vi "Measure_Synthetic_Jet.vi"(3 "Mode":T1=enum."Run VI", 5 "Traverse line In":T3={"Start X"=0.0, "Start Y"=0.0, "Start Z"=0.0, "End X"=nan, "End Y"=nan, "End Z"=nan, "nPoints"=5, "Spacing"=enum."Linear", "Filename"=path "C:/EnFlo_Data_Local/2013/Aero_Tunnel/Nick_Martin/Results/01-2013/QA_test_I.xls", "Tunnel Speed"=nan, "Averaging time (mins)"=0.08, "Extra Commands"="", "Carrier_1 Q (l/min)"=nan, "Carrier_2 Q (l/min)"=5.0, "Trace Gas Concentration (%)"=nan, "Specific Arguments"="Measure_Synthetic_Jet.vi; 200; 1000; 100", "Comments"="", "Row No"=0, "Row Type Selector"=enum."Run VI Named:", "EstCompl"="17:12  07-01-2013", "Row Duration (mins)"=4.483248000000001, "nValidPoints"=5, "Meas Setup File"="LDA_SJ_A.xls"} {"Carrier_2 Q (l/min)" format="%#.2f"; "Row Duration (mins)" format="%#.1f"; "Row No" min=0; "Trace Gas Concentration (%)" min=0.0 format="%#_4f"; "Carrier_1 Q (l/min)" format="%#.4f"; "Start X" format="%#.2f"; "Start Y" format="%#.2f"; "Start Z" format="%#.2f"; "End X" format="%#.2f"; "End Y" format="%#.2f"; "End Z" format="%#.2f"; "Tunnel Speed" format="%#.2f"; "Averaging time (mins)" min=0.0 format="%#.2f"}) -> (0 "Error Message":string, 1 "Status":T2, 2 "Traverse line Out":T3={"Start X"=0.0, "Start Y"=0.0, "Start Z"=0.0, "End X"=nan, "End Y"=nan, "End Z"=nan, "nPoints"=5, "Spacing"=enum."Linear", "Filename"=path "C:/EnFlo_Data_Local/2013/Aero_Tunnel/Nick_Martin/Results/01-2013/QA_test_I.xls", "Tunnel Speed"=nan, "Averaging time (mins)"=0.08, "Extra Commands"="", "Carrier_1 Q (l/min)"=nan, "Carrier_2 Q (l/min)"=5.0, "Trace Gas Concentration (%)"=nan, "Specific Arguments"="Measure_Synthetic_Jet.vi; 200; 1000; 100", "Comments"="", "Row No"=0, "Row Type Selector"=enum."Run VI Named:", "EstCompl"="17:12  07-01-2013", "Row Duration (mins)"=4.483248000000001, "nValidPoints"=5, "Meas Setup File"="LDA_SJ_A.xls"} {"Carrier_2 Q (l/min)" format="%#.2f"; "Row Duration (mins)" format="%#.1f"; "Row No" min=0; "Trace Gas Concentration (%)" min=0.0 format="%#_4f"; "Carrier_1 Q (l/min)" format="%#.4f"; "Start X" format="%#.2f"; "Start Y" format="%#.2f"; "Start Z" format="%#.2f"; "End X" format="%#.2f"; "End Y" format="%#.2f"; "End Z" format="%#.2f"; "Tunnel Speed" format="%#.2f"; "Averaging time (mins)" min=0.0 format="%#.2f"})   [LabVIEW 2022 SP3]
uses:
  <vilib>/Analysis/NI_AALBase.lvlib
  Globals/Synthetic_jet_global.vi
  Controls/Setup.ctl
  Controls/Save_Data.ctl
  Globals/Extra_Commands_Global.vi
  ADAM Client/Sub VIs/ADAM Controls/Update_scan_value.ctl
  <vilib>/Analysis/1siggen.llb/Ramp Pattern by Samples.vi
  Globals/Meas_global.vi
  Controls/User_Specific_mode.ctl
  Gen Trav/Multi_Run_Status.ctl
  Gen Trav/Spacing.ctl
  Controls/Multi_run_mode.ctl
  Gen Trav/Traverse_cluster.ctl
panel:
  in  "Enter SJ Data?":bool=TRUE
  in  "Stop Button":bool
  out "Last Meas Point":bool=TRUE
  out "Data":cluster{"Ramp Pattern":dbl[], dbl[]}[](graph)
  in  "Channels to Analyse":i32[](listbox)=[0]
  in  "VISA resource name":refnum<visa-resource-name>="USB0::0x0699::0x0347::C036837::INSTR"
  out "First Meas Point":bool=TRUE
  # "Check the Multirun in order to populate these Channels!"
  # "X           Y          Z"
  # "Start"
  # "End"
  # "X           Y          Z"
  # "Start"
  # "End"
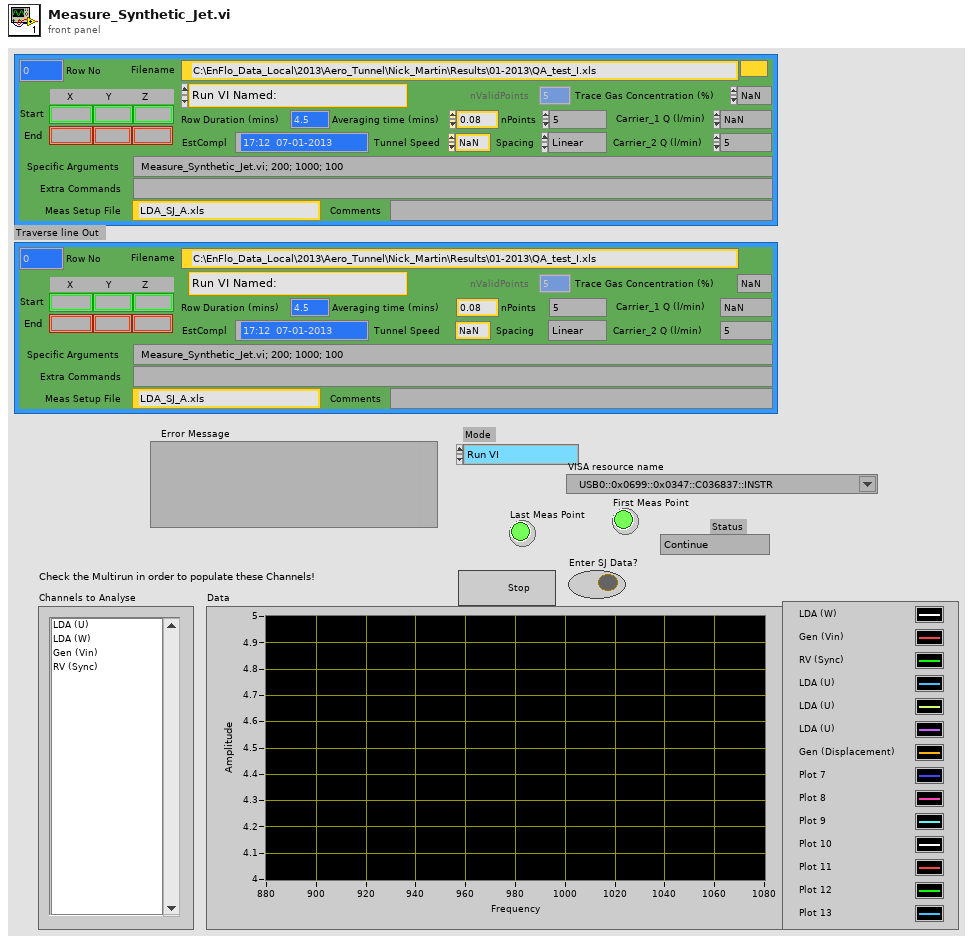
[diagram p1: front panel]
types:
  T1 = typedef "User_Specific_mode.ctl" = enum16{"Check VI only", "Run VI"}
  T2 = typedef "Multi_Run_Status.ctl" = enum16{"Continue", "Continue with Error", "Jump to Next Point", "Jump to Next Row", "Jump To Fall Back", "Terminate Run"}
  T3 = typedef "Traverse_cluster.ctl" = cluster{"Start X":sgl, "Start Y":sgl, "Start Z":sgl, "End X":sgl, "End Y":sgl, "End Z":sgl, "nPoints":i32, "Spacing":T4, "Filename":path, "Tunnel Speed":dbl, "Averaging time (mins)":dbl, "Extra Commands":string, "Carrier_1 Q (l/min)":dbl, "Carrier_2 Q (l/min)":dbl, "Trace Gas Concentration (%)":dbl, "Specific Arguments":string, "Comments":string, "Row No":i32, "Row Type Selector":T5, "EstCompl":string, "Row Duration (mins)":dbl, "nValidPoints":i32, "Meas Setup File":string}
  T4 = typedef "Spacing.ctl" = enum16{"Linear", "Log", "Gauss", "Specified", "N/A"}
  T5 = typedef "Multi_run_mode.ctl" = enum16{"Move Traverse Only", "Set Tunnel Speed Only", "Set Source Only", "Set Measurement Conditions", "Single Measurement", "Vertical Profile", "Lateral Profile", "Longitudinal Profile", "Multi-Axis Profile", "Explore Volume", "Auto Calibrate", "Meas Fast FID Bkgnd", "Check Beam Power", "Scanning Valve Measurement", "Run VI Named:", "Set ADAM Ch", "Wait (minutes)", "Send Message", "Synchronize With:", "Fall Back to this Row", "Turn Off Row Repeating", "Traverse 3D Volume", "Blank Row", "Jump to Fall Back Row"}
  T6 = typedef "Analysis_info_cluster.ctl" = cluster{"Colour":u32, "Inst type":T7, "Inst name":string, "Symbol":string, "Code name":string, "Extra Info":string, "Inst Array":T8, "Extra Titles":string[], "Extra Values":string[], "U":dbl, "u^2":dbl, "u^3":dbl, "u^4":dbl, "Skew_u":dbl, "Kurt_u":dbl, "Sd Error in Mean":dbl, "% u'/U":dbl, "X":dbl, "Y":dbl, "Z":dbl, "Timescale integral Estimate":dbl, "Sd Error in Variance":dbl, "Calib File":path, "Calib Constants":dbl[], "Output Position":bool, "Stats":enum16{"None", "Basic", "Full"}, "Av Sampling Rate":dbl, "Av No of Samples":dbl, "Total Meas Time (s)":dbl, "ADAM Ch Name":string, "Max value":dbl, "Min value":dbl, "Req Sample Rate Hz":dbl, "Sync Delay Time (s)":dbl, "Ch No":i16, "Device":string, "Use Latest Calib":bool, "Port":string, "Metadata Ch Names":string[], "Metadata Ch Values":string[], "Label":string}
  T7 = typedef "Inst_type.ctl" = enum16{"Raw voltage", "Raw with zero offsetting", "Propeller anemometer", "Pressure Transducer", "Pitot-static tube", "Hot wire", "Cross wire 1", "Cross wire 2", "Generic Linear", "Generic Polynomial", "Generic BackPoly", "Fast FID", "Thermocouple", "Cold wire", "Pulsed Wire", "LDA Vel", "LDA Tran time", "LDA Arr time", "Microphone"}
  T8 = typedef "Instrument_Array.ctl" = enum16{"PWA", "LDA", "Analogue"}
  T9 = typedef "Save_Data.ctl" = enum16{"Save No Data", "Save Data"}
  T10 = typedef "Setup.ctl" = enum16{"Run Program", "Show Setup", "Save Current Setup", "Setup Front Panel"}
  T11 = typedef "SJ_Data_Cluster.ctl" = cluster{"Do (mm)":dbl, "Dc (mm)":dbl, "Ho (mm)":dbl, "Hc (mm)":dbl, "K":dbl, "beta":dbl, "Vc (m^3)":dbl, "Vo (m^3)":dbl}
  T12 = typedef "Update_scan_value.ctl" = cluster{"Channel Name":string, "New Value":dbl, "!Auto_Off":bool}
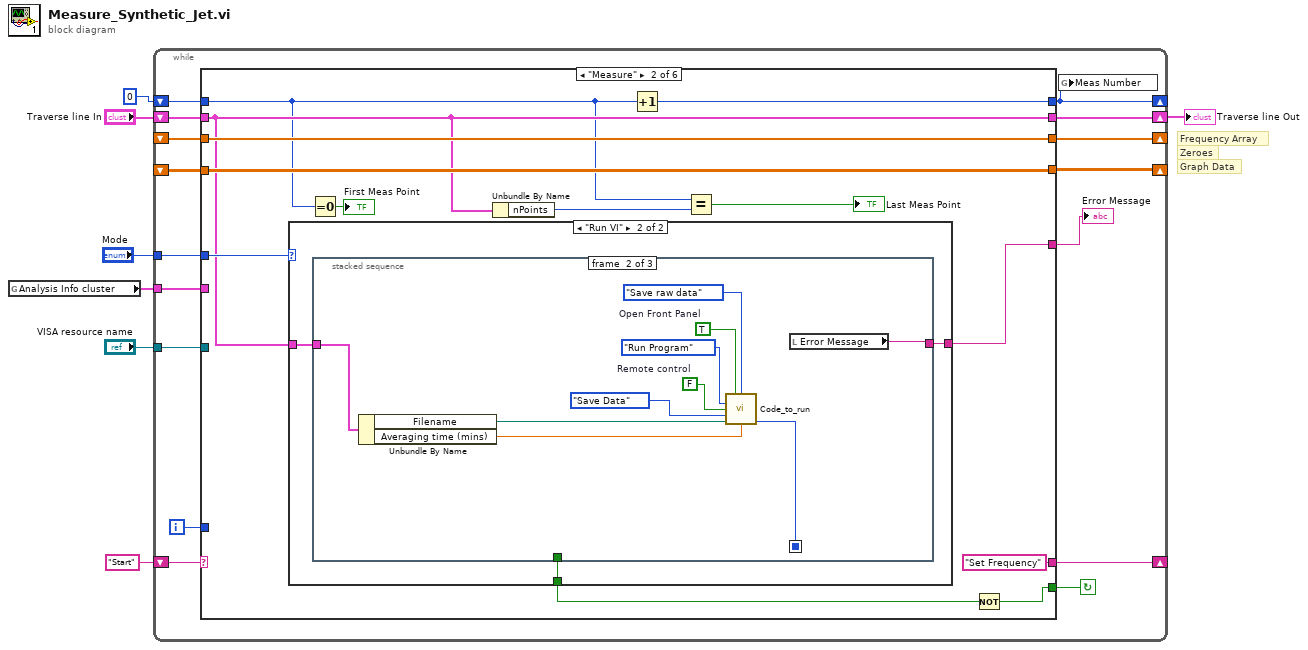
[diagram p0: block diagram]
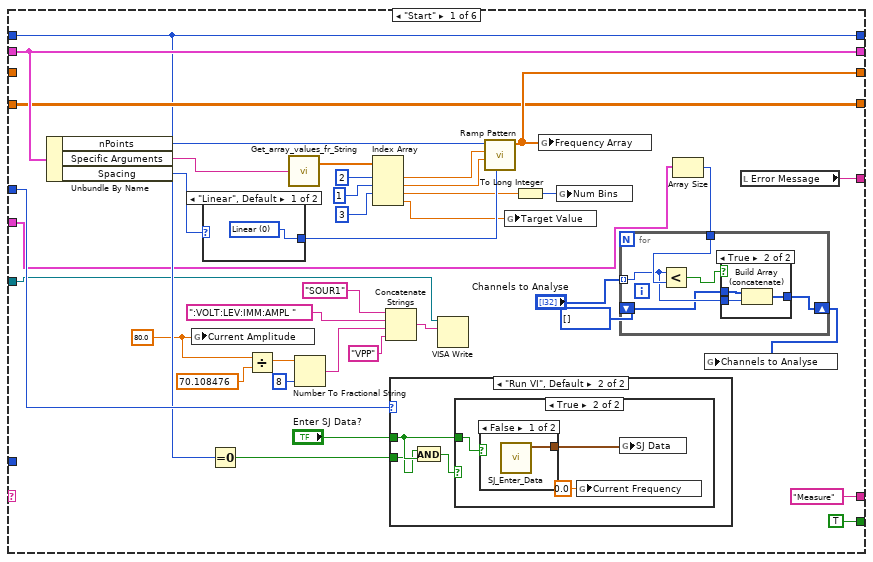
[diagram p2: hidden frame]
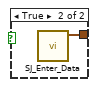
[diagram p6: hidden frame]
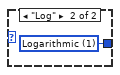
[diagram p7: hidden frame]
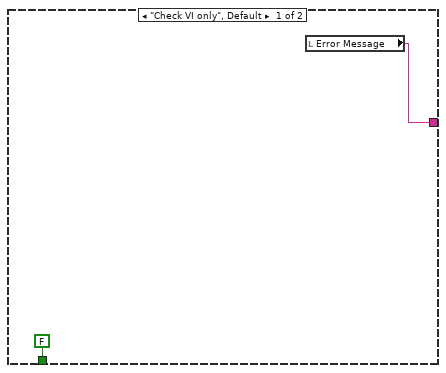
[diagram p8: hidden frame]
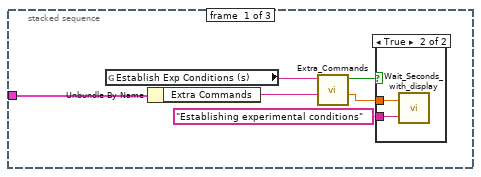
[diagram p9: hidden frame]
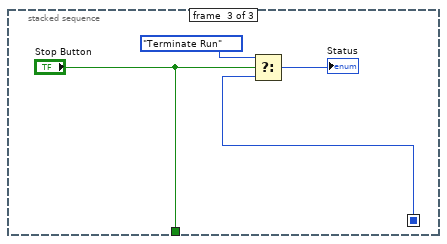
[diagram p11: hidden frame]
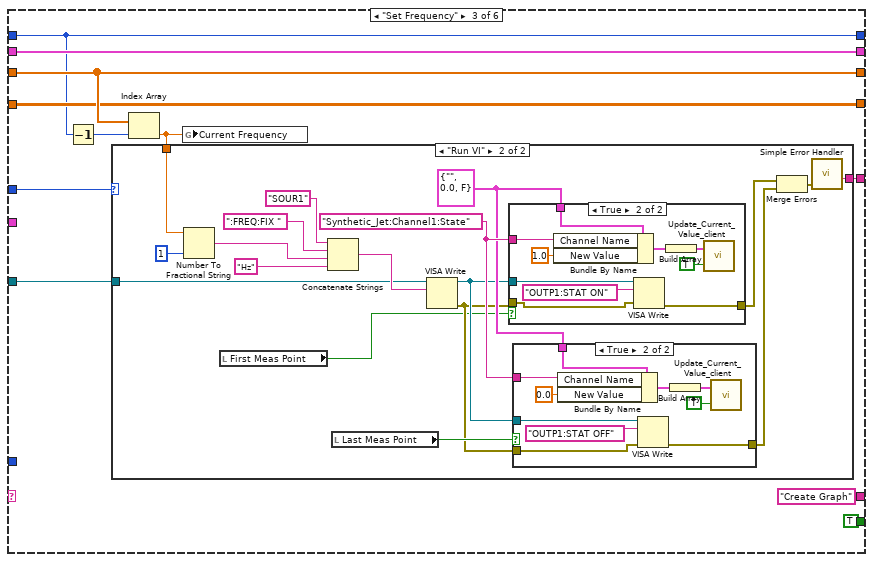
[diagram p12: hidden frame]
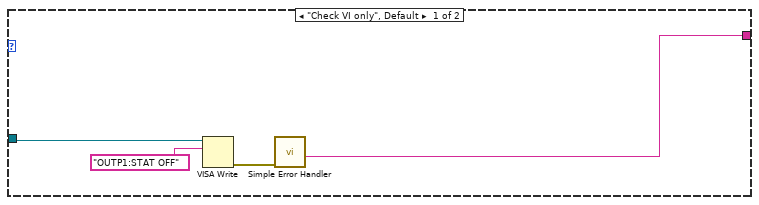
[diagram p13: hidden frame]
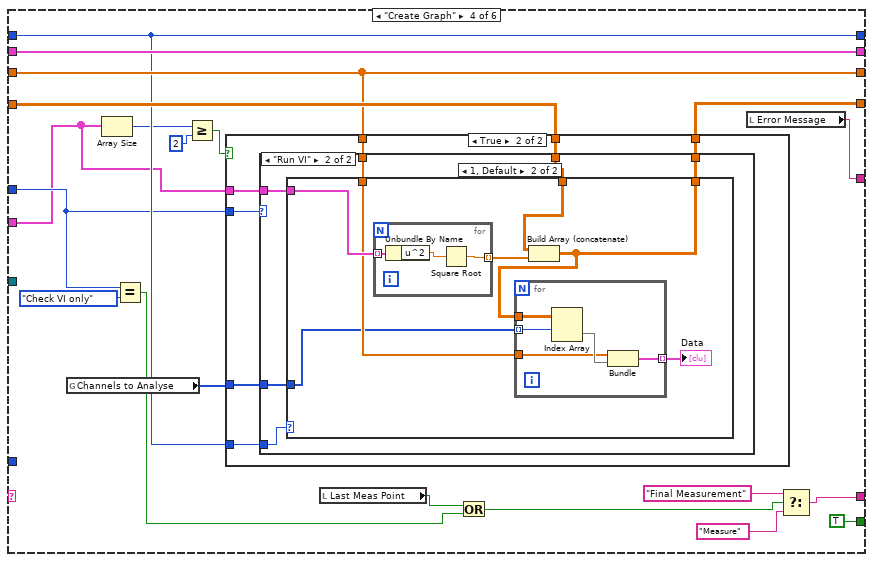
[diagram p16: hidden frame]
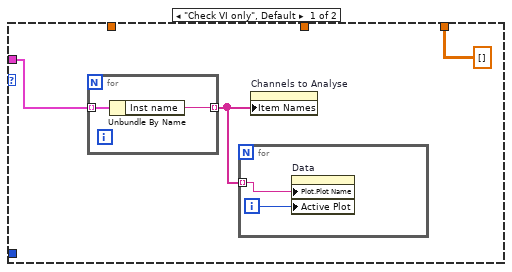
[diagram p18: hidden frame]
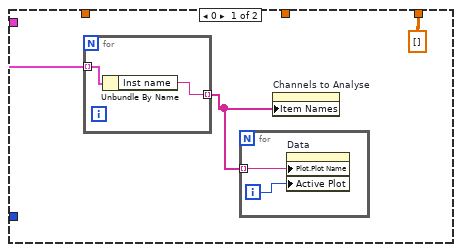
[diagram p19: hidden frame]
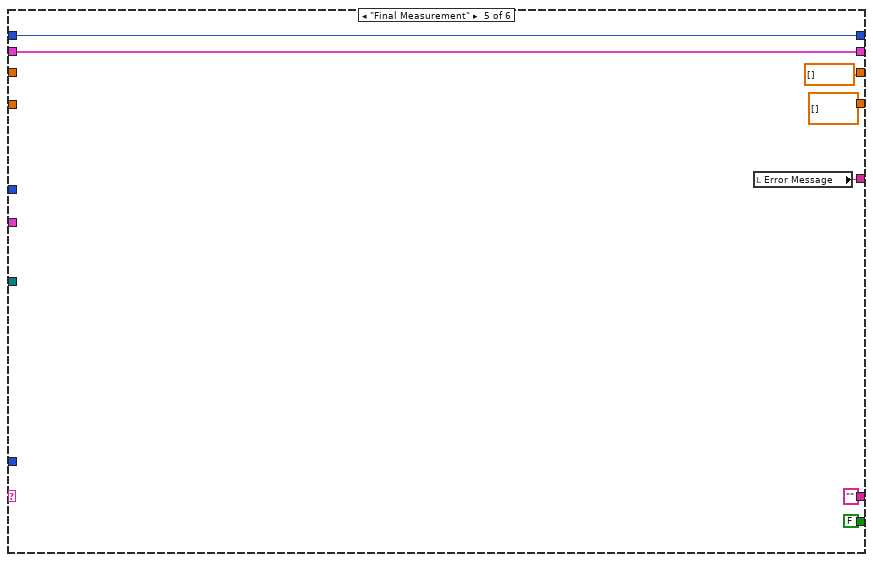
[diagram p20: hidden frame]
diagram:
  # "Graph Data"
  # "Zeroes"
  # "Frequency Array"
  n1 = global read "Meas_global.vi" "Analysis Info cluster"() -> (w1:T6[])
  n2 = while {
    shift-right: [w21] -> _
    shift-left: "Start" -> [w20]
    shift-right: [w19] -> w5
    shift-left: "Traverse line In" -> [w23]
    shift-right: [w18] -> _
    shift-left: _ -> [w17]
    tunnel: "Mode" -> [w16]
    tunnel: "VISA resource name" -> [w14]
    shift-right: [w13] -> _
    shift-left: _ -> [w12]
    shift-right: [w9] -> _
    shift-left: 0 -> [w10]
    tunnel: w1 -> [w8]
    i -> [w15]
    stop <- w22 continue-if-true
    n3 = case shown="\"Measure\"" w20 {
      selector: w20 -> [_ _ _ _ _ w250]
      tunnel: w23 -> [w59 w87 w129 w195 w243 w258]
      tunnel: [TRUE w81 TRUE TRUE ("Last Meas Point") FALSE ("Last Meas Point") FALSE] -> w22
      tunnel: ["Measure" "Set Frequency" "Create Graph" w189 "" ""] -> w21
      tunnel: [w59 w87 w129 w195 w243 w258] -> w19
      tunnel: [w47 w92 w128 w192 dbl[] [] ("Ramp Pattern") w249] -> w18
      tunnel: w17 -> [_ w92 w128 w192 _ w249]
      tunnel: w16 -> [w48 w91 w124 w185 _ _]
      tunnel: w15 -> [_ _ _ _ _ _]
      tunnel: w14 -> [w33 _ w125 _ _ _]
      tunnel: [w46 w90 w123 w194 dbl[][] [] w248] -> w13
      tunnel: w12 -> [w46 w90 w123 w193 _ w248]
      tunnel: [w45 w89 w122 w191 w242 w247] -> w11
      tunnel: [w41 w85 w121 w186 w239 w246] -> w9
      tunnel: w10 -> [w41 w83 w121 w186 w239 w246]
      tunnel: w8 -> [w28 _ _ w176 _ _]
      frame "Start" {
        w30 = 80.0 ("number")
        n4 = Unbundle By Name(w59) -> ("nPoints"=w58:i32, "Specific Arguments"=w55:string, "Spacing"=w57:T4)
        n5 = global write "Synthetic_jet_global.vi" "Current Amplitude"(w30) -> ()
        n6 = case shown="\"Linear\", Default" w57 {
          tunnel: [w79 w80] -> w56
          frame "Linear", Default {
            w79 = u16 0 items=["Linear", "Logarithmic"] ("type")
          }
          frame "Log" {
            w80 = u16 1 items=["Linear", "Logarithmic"] ("type")
          }
        }
        n7 = Equal To 0?(x=w41) -> (x = 0?=w49:bool)
        n8 = Divide(x=w30, y=70.108476) -> (x/y=w32:dbl)
        n9 = call "Get_array_values_fr_String.vi"("String Value"=w55) -> ("Numeric Array"=w54:dbl[])  [unwired: 1 out]
        n10 = Number To Fractional String(number=w32, precision (6)=i16 8) -> (F-format string=w35:string)  [unwired: 2 in]
        n11 = Index Array(array=w54, index #1=2 ("index"), index #2=1 ("index"), index #3=3 ("index")) -> (element #1=w51:dbl, element #2=w50:dbl, element #3=w43:dbl, element #4=w40:dbl)  [unwired: 1 in]
        n12 = Concatenate Strings("SOUR1" ("string"), ":VOLT:LEV:IMM:AMPL " ("string"), w35, "VPP" ("string")) -> (w36:string)
        n13 = case shown="\"Run VI\", Default" w48 {
          tunnel: w49 -> [_ w72]
          tunnel: "Enter SJ Data?" -> [_ w73]
          frame "Check VI only" {
          }
          frame "Run VI", Default {
            n14 = And(x=w72, y=w73) -> (x .and. y?=w71:bool)
            n15 = case shown="True" w71 {
              tunnel: w73 -> [_ w75]
              frame False {
              }
              frame True {
                n16 = case shown="False" w75 {
                  tunnel: [w77 w78] -> w74
                  frame False {
                    n17 = call "SJ_Enter_Data.vi"() -> ("SJ Data"=w77:T11)  [unwired: 11 in]
                  }
                  frame True {
                    n18 = call "SJ_Enter_Data.vi"() -> ("SJ Data"=w78:T11)  [unwired: 11 in]
                  }
                }
                n19 = global write "Synthetic_jet_global.vi" "Current Frequency"(0.0 ("Current Frequency")) -> ()
                n20 = global write "Synthetic_jet_global.vi" "SJ Data"(w74) -> ()
              }
            }
          }
        }
        n21 = VISA Write(VISA resource name=w33, write buffer=w36) -> ()  [unwired: 1 in, 3 out]
        n22 = call-poly <vilib>:"Ramp Pattern.vi"("type"=w56, "start"=w50, "end"=w51, "samples"=w58) -> ("Ramp Pattern"=w47:dbl[])  [unwired: 6 in, 1 out]
        n23 = global write "Synthetic_jet_global.vi" "Target Value"(w40) -> ()
        n24 = To Long Integer(number=w43) -> (32bit integer=w42:i32)
        n25 = global write "Synthetic_jet_global.vi" "Frequency Array"(w47) -> ()
        n26 = global write "Synthetic_jet_global.vi" "Num Bins"(w42) -> ()
        n27 = Array Size(array=w28) -> (size(s)=w29:i32)
        n28 = for {
          tunnel: w29 -> [w66]
          tunnel: "Channels to Analyse" -> [w64] mode=indexing
          shift-right: [w63] -> w26
          shift-left: i32[] [] -> [w62]
          n29 = Less?(x=w64, y=w66) -> (x < y?=w65:bool)
          n30 = case shown="True" w65 {
            tunnel: w64 -> [_ w70]
            tunnel: [w67 w69] -> w63
            tunnel: w62 -> [w67 w68]
            frame False {
            }
            frame True {
              n31 = Build Array (concatenate)(w68, w70) -> (w69:i32[])
            }
          }
        }
        n32 = global write "Synthetic_jet_global.vi" "Channels to Analyse"(w26) -> ()
        n33 = local read "Error Message"() -> (w45:string)
      }
      frame "Measure" {
        n34 = case shown="\"Run VI\"" w91 {
          tunnel: w87 -> [_ w98]
          tunnel: [w95 w97] -> w89
          tunnel: [FALSE ("Stop Button") w96] -> w82
          frame "Check VI only", Default {
            n35 = local read "Error Message"() -> (w95:string)
          }
          frame "Run VI" {
            n36 = stacked-sequence {
              seq-local: [_ w107 _] -> [_ _ w118]
              tunnel: w98 -> [w99 w112 _]
              tunnel: [_ w109 _] -> w97
              tunnel: [_ _ "Stop Button"] -> w96
              frame #0 {
                n37 = global read "Extra_Commands_Global.vi" "Establish Exp Conditions (s)"() -> (w102:string)
                n38 = Unbundle By Name(w99) -> ("Extra Commands"=w100:string)
                n39 = call "Extra_Commands.vi"("String to Search"=w100, "Command"=w102) -> ("Numeric Value"=w101:dbl, "Command Found"=w103:bool)  [unwired: 2 in, 2 out]
                n40 = case shown="True" w103 {
                  tunnel: w101 -> [_ w106]
                  tunnel: "Establishing experimental conditions" ("Message") -> [_ w105]
                  frame False {
                  }
                  frame True {
                    n41 = call "Wait_Seconds_with_display.vi"("Message"=w105, "Seconds to wait"=w106) -> ()  [unwired: 1 in, 1 out]
                  }
                }
              }
              frame #1 {
                w114 = TRUE  # Open Front Panel
                w113 = FALSE  # Remote control
                n42 = Unbundle By Name(w112) -> ("Filename"=w111:path, "Averaging time (mins)"=w108:dbl)
                n43 = call "Code_to_run.vi"("Open Front Panel"=w114, "Raw data option"=enum16{"Save raw data", "Raw data not saved"}."Save raw data", "setup"=Setup."Run Program", "Remote control"=w113, "File"=Save_Data."Save Data", "Results Filename"=w111, "Averaging time (min)"=w108) -> ("Status"=w107:T2)  [unwired: 5 in, 3 out]
                n44 = local read "Error Message"() -> (w109:string)
              }
              frame #2 {
                n45 = Select(t=Multi_Run_Status."Terminate Run", s="Stop Button", f=w118) -> (s? t:f=→"Status":T2)
              }
            }
          }
        }
        n46 = Equal To 0?(x=w83) -> (x = 0?=→"First Meas Point":bool)
        n47 = Unbundle By Name(w87) -> ("nPoints"=w86:i32)
        n48 = Increment(x=w83) -> (x+1=w85:i32)
        n49 = Equal?(x=w83, y=w86) -> (x = y?=→"Last Meas Point":bool)
        n50 = Not(x=w82) -> (.not. x?=w81:bool)
      }
      frame "Set Frequency" {
        n51 = Decrement(x=w121) -> (x-1=w127:i32)
        n52 = Index Array(array=w128, index=w127) -> (element=w126:dbl)
        n53 = case shown="\"Run VI\"" w124 {
          tunnel: w126 -> [_ w145]
          tunnel: w125 -> [w134 w144]
          tunnel: [w132 w141] -> w122
          frame "Check VI only", Default {
            n54 = VISA Write(VISA resource name=w134, write buffer="OUTP1:STAT OFF") -> (error out=w133:errorcluster)  [unwired: 1 in, 2 out]
            n55 = call <vilib>:"Simple Error Handler.vi"("error in (no error)"=w133) -> ("source out"=w132:string)  [unwired: 4 in, 4 out]
          }
          frame "Run VI" {
            w146 = T12 {"Channel Name"="", "New Value"=0.0, "!Auto_Off"=FALSE} ("Update Scan Value Cluster")
            w147 = "Synthetic_Jet:Channel1:State" ("write buffer")
            n56 = Number To Fractional String(number=w145, precision (6)=i16 1) -> (F-format string=w151:string)  [unwired: 2 in]
            n57 = local read "First Meas Point"() -> (w136:bool)
            n58 = Concatenate Strings("SOUR1", ":FREQ:FIX " ("string"), w151, "Hz" ("string")) -> (w153:string)
            n59 = local read "Last Meas Point"() -> (w143:bool)
            n60 = VISA Write(VISA resource name=w144, write buffer=w153) -> (VISA resource name out=w142:refnum<visa-resource-name>, error out=w137:errorcluster)  [unwired: 1 in, 1 out]
            n61 = case shown="True" w136 {
              tunnel: w147 -> [_ w170]
              tunnel: w146 -> [_ w169]
              tunnel: w142 -> [_ w168]
              tunnel: [w165 w167] -> w138
              tunnel: w137 -> [w165 w166]
              frame False {
              }
              frame True {
                n62 = Bundle By Name(cluster=w169, "Channel Name"=w170, "New Value"=1.0) -> (w173:T12)
                n63 = VISA Write(VISA resource name=w168, write buffer="OUTP1:STAT ON", error in (no error)=w166) -> (error out=w167:errorcluster)  [unwired: 2 out]
                n64 = Build Array(w173) -> (w172:T12[])
                n65 = call "Update_Current_Value_client.vi"("Don't Bother with check?"=TRUE, "Update array in"=w172) -> ()
              }
            }
            n66 = case shown="True" w143 {
              tunnel: w147 -> [_ w159]
              tunnel: w146 -> [_ w158]
              tunnel: w142 -> [_ w157]
              tunnel: [w154 w156] -> w139
              tunnel: w137 -> [w154 w155]
              frame False {
              }
              frame True {
                n67 = Bundle By Name(cluster=w158, "Channel Name"=w159, "New Value"=0.0) -> (w162:T12)
                n68 = VISA Write(VISA resource name=w157, write buffer="OUTP1:STAT OFF", error in (no error)=w155) -> (error out=w156:errorcluster)  [unwired: 2 out]
                n69 = Build Array(w162) -> (w161:T12[])
                n70 = call "Update_Current_Value_client.vi"("Don't Bother with check?"=TRUE, "Update array in"=w161) -> ()
              }
            }
            n71 = Merge Errors(w138, w139) -> (w140:errorcluster)
            n72 = call <vilib>:"Simple Error Handler.vi"("error in (no error)"=w140) -> ("source out"=w141:string)  [unwired: 4 in, 4 out]
          }
        }
        n73 = global write "Synthetic_jet_global.vi" "Current Frequency"(w126) -> ()
      }
      frame "Create Graph" {
        n74 = global read "Synthetic_jet_global.vi" "Channels to Analyse"() -> (w177:i32[])
        n75 = Array Size(array=w176) -> (size(s)=w178:i32)
        n76 = Equal?(x=w185, y=User_Specific_mode."Check VI only") -> (x = y?=w182:bool)
        n77 = Greater Or Equal?(x=w178, y=2 ("x")) -> (x >= y?=w180:bool)
        n78 = case shown="True" w180 {
          tunnel: w176 -> [_ w203]
          tunnel: [w196 w202] -> w194
          tunnel: w193 -> [w196 w201]
          tunnel: w192 -> [_ w200]
          tunnel: w186 -> [_ w199]
          tunnel: w185 -> [_ w198]
          tunnel: w177 -> [_ w197]
          frame False {
          }
          frame True {
            n79 = case shown="\"Run VI\"" w198 {
              tunnel: w203 -> [w206 w216]
              tunnel: w199 -> [_ w215]
              tunnel: [dbl[][] [] w214] -> w202
              tunnel: w201 -> [_ w213]
              tunnel: w200 -> [_ w212]
              tunnel: w197 -> [_ w211]
              frame "Check VI only", Default {
                n80 = for {
                  tunnel: w206 -> [w210] mode=indexing
                  tunnel: [w209] -> w204 mode=indexing
                  n81 = Unbundle By Name(w210) -> ("Inst name"=w209:string)
                }
                n82 = for {
                  tunnel: w204 -> [w208] mode=indexing
                  i -> [w207]
                  n83 = property on="Data" class="XYGraph (strict)"("Plot.Plot Name"=w208, "Active Plot"=w207) -> ()  [unwired: 2 in, 2 out]
                }
                n84 = property on="Channels to Analyse" class="LstBox (strict)"("Item Names"=w204) -> ()  [unwired: 2 in, 2 out]
              }
              frame "Run VI" {
                n85 = case shown="1, Default" w215 {
                  tunnel: w216 -> [w219 w230]
                  tunnel: [dbl[][] [] w227] -> w214
                  tunnel: w213 -> [_ w228]
                  tunnel: w212 -> [_ w226]
                  tunnel: w211 -> [_ w224]
                  frame 0 {
                    n86 = for {
                      tunnel: w219 -> [w223] mode=indexing
                      tunnel: [w222] -> w217 mode=indexing
                      n87 = Unbundle By Name(w223) -> ("Inst name"=w222:string)
                    }
                    n88 = for {
                      tunnel: w217 -> [w221] mode=indexing
                      i -> [w220]
                      n89 = property on="Data" class="XYGraph (strict)"("Plot.Plot Name"=w221, "Active Plot"=w220) -> ()  [unwired: 2 in, 2 out]
                    }
                    n90 = property on="Channels to Analyse" class="LstBox (strict)"("Item Names"=w217) -> ()  [unwired: 2 in, 2 out]
                  }
                  frame 1, Default {
                    n91 = for {
                      tunnel: w230 -> [w238] mode=indexing
                      tunnel: [w236] -> w229 mode=indexing
                      n92 = Unbundle By Name(w238) -> ("u^2"=w237:dbl)
                      n93 = Square Root(x=w237) -> (sqrt(x)=w236:dbl)
                    }
                    n94 = Build Array (concatenate)(w228, w229) -> (w227:dbl[][])
                    n95 = for {
                      tunnel: w227 -> [w235]
                      tunnel: w224 -> [w231] mode=indexing
                      tunnel: w226 -> [w233]
                      tunnel: [w232] -> w225 mode=indexing
                      n96 = Index Array(array=w235, index (row)=w231) -> (element=w234:dbl[])  [unwired: 1 in]
                      n97 = Bundle("Ramp Pattern"=w233, w234) -> (w232:cluster{"Ramp Pattern":dbl[], dbl[]})  [unwired: 1 in]
                    }
                    "Data" <- w225
                  }
                }
              }
            }
          }
        }
        n98 = local read "Last Meas Point"() -> (w183:bool)
        n99 = Or(x=w183, y=w182) -> (x .or. y?=w181:bool)
        n100 = local read "Error Message"() -> (w191:string)
        n101 = Select(t="Final Measurement", s=w181, f="Measure") -> (s? t:f=w189:string)
      }
      frame "Final Measurement" {
        n102 = local read "Error Message"() -> (w242:string)
      }
      frame "No Match", Default {
        n103 = Current VI's Path() -> (path=w255:path)
        n104 = Format Into String(format string="The Case\"%s\" was not Matched\nin VI named\n'%s\"" ("Format String"), w250, w255) -> (resulting string=w252:string)  [unwired: 2 in, 1 out]
        n105 = One Button Dialog(message=w252, button name ("OK")="STOP") -> (true=w254:bool)
        n106 = Stop(stop? (T)=w254) -> ()
        n107 = local read "Error Message"() -> (w247:string)
      }
    }
    "Error Message" <- w11
    n108 = global write "Synthetic_jet_global.vi" "Meas Number"(w9) -> ()
  }
  "Traverse line Out" <- w5
